vi "Estimate All Positions - Swarm Method (copy).vi"(0 "TagArray In":refnum<class "Tag.lvclass">[](array[class]), 1 "AllTagDistancesArray":T2(array[cluster]), 2 "AltTDA":T2(array[cluster]), 3 "Werkpunten":T5(array[cluster]), 5 "AnchorsArray":refnum<class "Anchor.lvclass">[](array[class]), 7 "error in (no error)":errorcluster) -> (13 "error out":errorcluster, 15 "Solution Vector":dbl[](array[numeric]) format="%.2f", 17 "SwarmOutputArray":T4(array[cluster]))   [LabVIEW 2014]
uses:
  Tag.lvclass
  Anchor/Anchor.lvclass
  <vilib>/Analysis/Matrix/Datatypes/RealMatrix.ctl
  <vilib>/Analysis/baseanly.llb/Matrix Type of Inverse Matrix.ctl
  <vilib>/Analysis/7linalg.llb/Solve Linear Equations (single right hand).vi
  <vilib>/Analysis/baseanly.llb/Solve Linear Equations By Cholesky.vi
  <vilib>/Analysis/baseanly.llb/Real Matrix to Compact Array.vi
  <vilib>/Analysis/baseanly.llb/Real Compact Tri-Matrix Linear Eqs.vi
  <vilib>/Analysis/Matrix/Numeric/Conversions/Array To Matrix - RA2.vi
  <vilib>/Analysis/7linalg.llb/Solve Linear Eqs (General).vi
  <vilib>/Analysis/7linalg.llb/Solve Linear Eqs (Gen, single right hand).vi
  <vilib>/Analysis/NI_AALPro.lvlib
  <vilib>/Analysis/NI_AALBase.lvlib
  <vilib>/Analysis/Matrix/NI_Matrix.lvlib
panel:
  out "fSwarmOutputArray":T1(array[cluster])
  out "RealSolutionVector":dbl[](array[numeric])
  out "Solution Vector AnchorToTag":dbl[](array[numeric]) format="%.2f"
  out "Solution Vector TagToTag":dbl[](array[numeric]) format="%.2f"
  out "Known Vector 3":T3
  out "Known Vector 2":T3
  out "Known Vector 1":T3
  out "Input Matrix 2":T3
  out "Input Matrix 1":T3
  out "Results Real":T3
  out "Input Matrix 3":T3
  out "# tags":i32=22
  out "Tag To":i32
  out "TagIDFrom":dbl format="%.2f"
  # "Output Indicators"
  # "Input Controls"
  # "Error Control"
  # "Error Indicator"
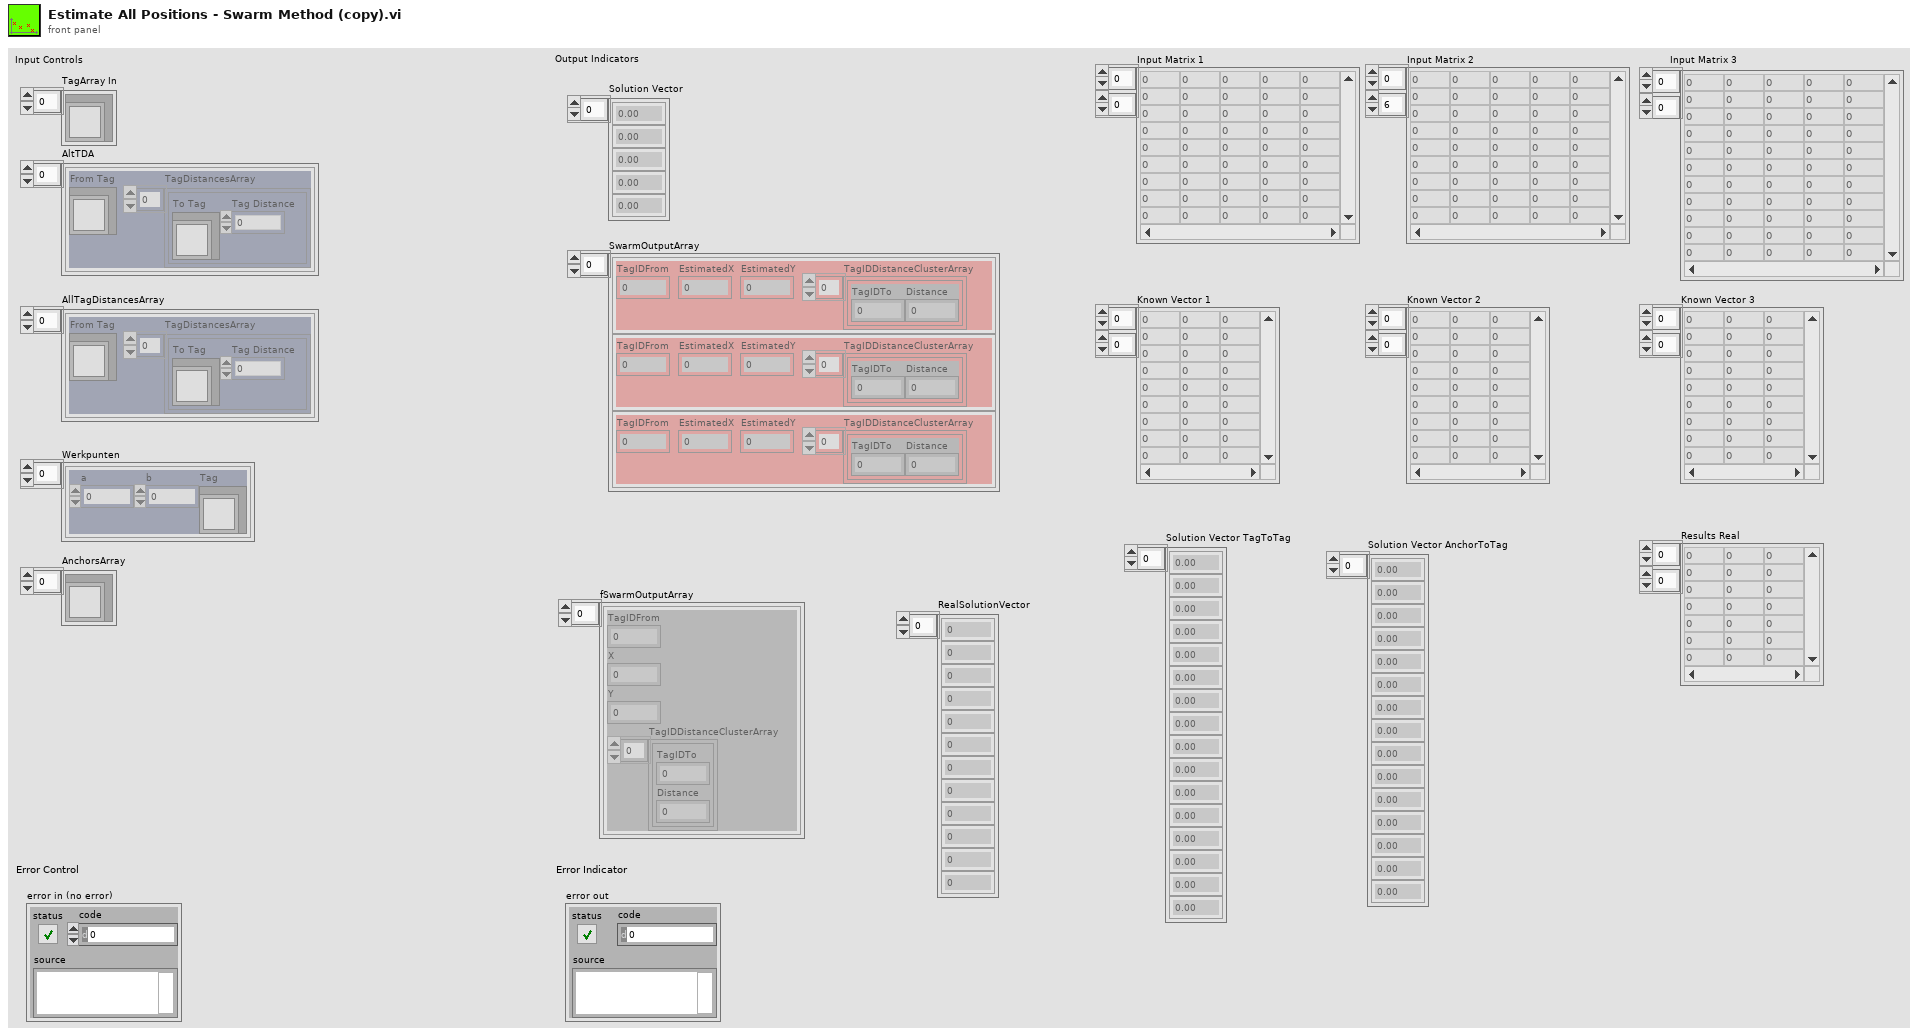
[diagram p1: front panel]
types:
  T1 = cluster{"TagIDFrom":dbl, "X":dbl, "Y":dbl, "TagIDDistanceClusterArray":cluster{"TagIDTo":dbl, "Distance":dbl}[]}[]
  T2 = cluster{"From Tag":refnum<class "Tag.lvclass">, "TagDistancesArray":cluster{"To Tag":refnum<class "Tag.lvclass">, "Tag Distance":dbl}[]}[]
  T3 = typedef "NI_Matrix.lvlib/RealMatrix.ctl" = dbl[][]
  T4 = cluster{"TagIDFrom":dbl, "EstimatedX":dbl, "EstimatedY":dbl, "TagIDDistanceClusterArray":cluster{"TagIDTo":dbl, "Distance":dbl}[]}[]
  T5 = cluster{"a":dbl, "b":dbl, "Tag":refnum<class "Tag.lvclass">}[]
  T6 = typedef "NI_AALBase.lvlib/Matrix Type of Inverse Matrix.ctl" = enum32{"General", "Positive Definite", "Lower Triangular", "Upper Triangular"}
  T7 = cluster{"From Tag":refnum<class "Tag.lvclass">, "TagDistancesArray":cluster{"To Tag":refnum<class "Tag.lvclass">, "Tag Distance":dbl}[]}
  T8 = cluster{"To Tag":refnum<class "Tag.lvclass">, "Tag Distance":dbl}[]
  T9 = cluster{"To Tag":refnum<class "Tag.lvclass">, "Tag Distance":dbl}
  T10 = cluster{"a":dbl, "b":dbl, "Tag":refnum<class "Tag.lvclass">}
  T11 = cluster{"TagID":dbl, dbl, dbl, "TagIDDistanceClusterArray":cluster{"TagIDTo":dbl, "Distance":dbl}[]}
  T12 = cluster{"TagID":dbl, "X":dbl, "Y":dbl, "TagIDDistanceClusterArray":cluster{"TagIDTo":dbl, "Distance":dbl}[]}[]
  T13 = cluster{"Tag.lvclass":refnum<class "Tag.lvclass">, "Distance":dbl}[]
  T14 = cluster{"TagIDFrom":dbl, "X":dbl, "Y":dbl, "TagIDDistanceClusterArray":cluster{"TagIDTo":dbl, "Distance":dbl}[]}
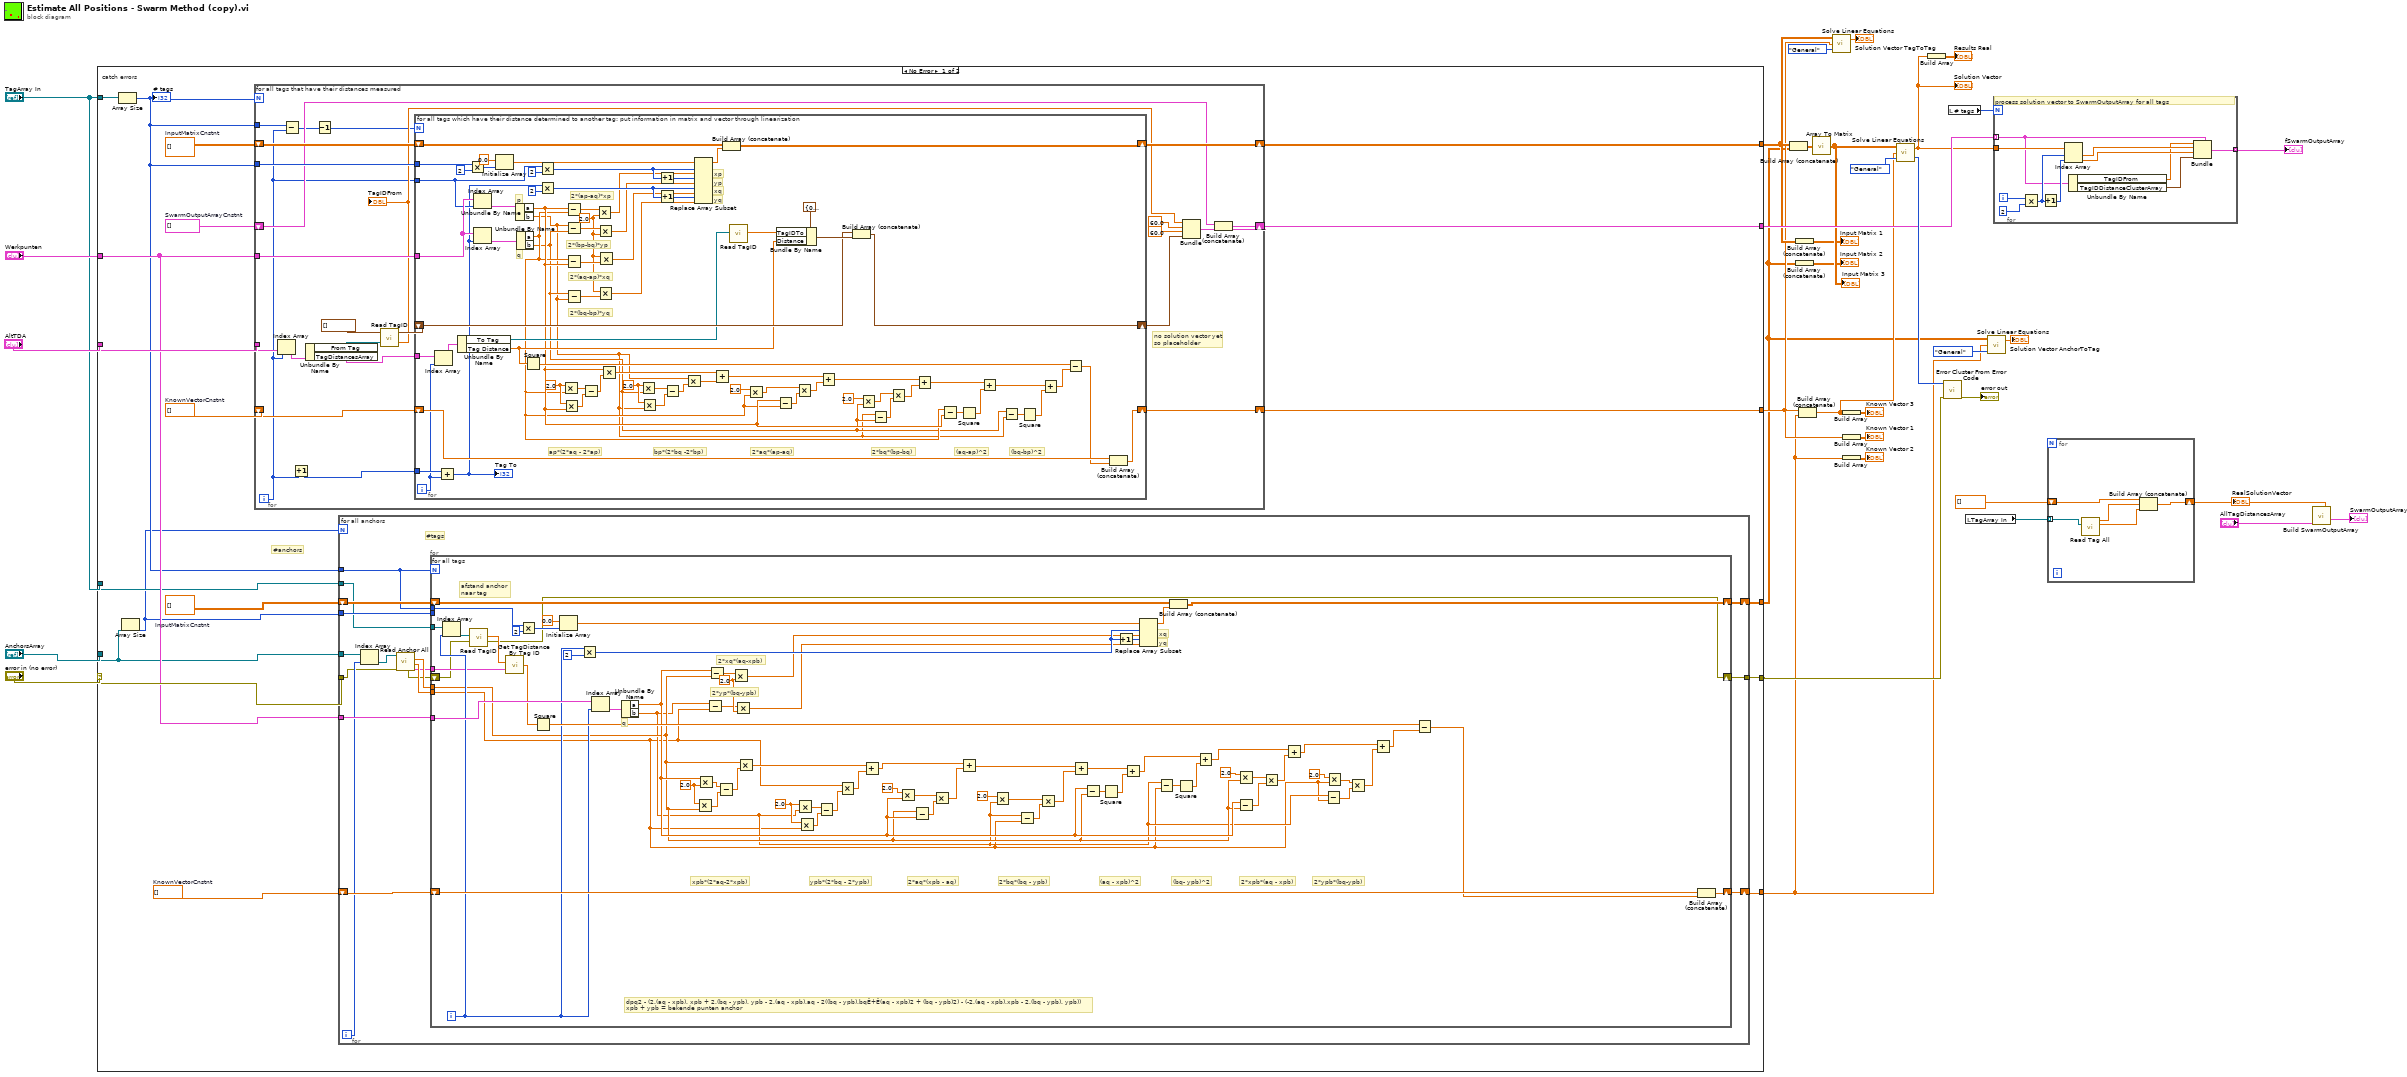
[diagram p0: block diagram]
diagram:
  n1 = case shown="No Error" "error in (no error)" {
    selector: "error in (no error)" -> [w48 w240]
    tunnel: [w53 _] -> w13
    tunnel: "Werkpunten" -> [w40 _]
    tunnel: "AnchorsArray" -> [w38 _]
    tunnel: [w51 _] -> w14
    tunnel: [w50 _] -> w9
    tunnel: [w49 _] -> w8
    tunnel: "TagArray In" -> [w43 _]
    tunnel: [w47 w240] -> w30
    tunnel: [w45 _] -> w28
    tunnel: "AltTDA" -> [w44 _]
    tunnel: "TagArray In" -> [w37 _]
    frame No Error {
      w41 = dbl[] []  # KnownVectorCnstnt
      w42 = dbl[][] []  # InputMatrixCnstnt
      w46 = T1 []  # SwarmOutputArrayCnstnt
      w52 = dbl[] []  # KnownVectorCnstnt
      w54 = dbl[][] []  # InputMatrixCnstnt
      # "#anchors"
      # "catch errors"
      n2 = Array Size(array=w43) -> (size(s)=w39:i32)
      "# tags" <- w39
      n3 = Array Size(array=w38) -> (size(s)=w36:i32)
      n4 = for {
        N: w39 -> [_]
        tunnel: w39 -> [w165]
        shift-right: [w162] -> w51
        shift-left: w54 -> [w163]
        tunnel: w39 -> [w161]
        tunnel: w40 -> [w160]
        shift-right: [w159] -> w53
        shift-left: w52 -> [w158]
        shift-right: [w153] -> w45
        shift-left: w46 -> [w154]
        tunnel: w44 -> [w147]
        i -> [w145]
        # "no solution vector yet\nso placeholder"
        # "for all tags that have their distances measured"
        n5 = Index Array "Index Array"(array=w147, index=w145) -> (element=w146:T7)
        n6 = Subtract(x=w165, y=w145) -> (x-y=w148:i32)
        n7 = Increment(x=w145) -> (x+1=w164:i32)
        n8 = Unbundle By Name(w146) -> ("From Tag"=w144:refnum<class "Tag.lvclass">, "TagDistancesArray"=w150:T8)
        n9 = Decrement(x=w148) -> (x-1=w143:i32)
        n10 = call "Read TagID.vi"("Tag in"=w144) -> ("TagID"=w149:dbl)  [unwired: 16 in, 2 out]
        "TagIDFrom" <- w149
        n11 = for {
          N: w143 -> [_]
          tunnel: w164 -> [w239]
          shift-right: [w238] -> w162
          shift-left: w163 -> [w232]
          tunnel: w161 -> [w234]
          tunnel: w160 -> [w216]
          tunnel: w145 -> [w215]
          shift-right: [w221] -> w159
          shift-left: w158 -> [w222]
          shift-right: [w217] -> w155
          shift-left: cluster{"TagIDTo":dbl, "Distance":dbl}[] [] ("TagIDDistanceClusterArray") -> [w218]
          tunnel: w150 -> [w211]
          i -> [w210]
          w192 = 2.0 ("x")
          w196 = 2.0 ("x")
          w199 = 2.0 ("y")
          # "(bq-bp)^2"
          # "(aq-ap)^2"
          # "2*bq*(bp-bq)"
          # "2*aq*(ap-aq)"
          # "bp*(2*bq -2*bp)"
          # "ap*(2*aq - 2*ap)"
          # "2*(bq-bp)*yq"
          # "2*(aq-ap)*xq"
          # "2*(bp-bq)*yp"
          # "2*(ap-aq)*xp"
          # "yq"
          # "xq"
          # "yp"
          # "xp"
          # "p"
          # "q"
          # "for all tags which have their distance determined to another tag: put information in matrix and vector through linearization"
          n12 = Index Array(array=w211, index=w210) -> (element=w209:T9)
          n13 = Add(x=w239, y=w210) -> (x+y=w212:i32)
          "Tag To" <- w212
          n14 = Unbundle By Name(w209) -> ("To Tag"=w213:refnum<class "Tag.lvclass">, "Tag Distance"=w208:dbl)
          n15 = Multiply(x=w234, y=2) -> (x*y=w237:i32)
          n16 = Index Array "Index Array"(array=w216, index=w215) -> (element=w230:T10)
          n17 = Index Array "Index Array"(array=w216, index=w212) -> (element=w229:T10)
          n18 = Initialize Array "Initialize Array"(0.0 ("element"), w237) -> (w231:dbl[])
          n19 = Unbundle By Name(w230) -> ("a"=w177:dbl, "b"=w169:dbl)
          n20 = Unbundle By Name(w229) -> ("a"=w176:dbl, "b"=w170:dbl)
          n21 = Square(x=w208) -> (x^2=w207:dbl)
          n22 = Multiply(x=w215, y=2) -> (x*y=w227:i32)
          n23 = Multiply(x=w212, y=2) -> (x*y=w224:i32)
          n24 = Multiply(x=w196, y=w176) -> (x*y=w197:dbl)
          n25 = Multiply(x=w196, y=w177) -> (x*y=w195:dbl)
          n26 = Subtract(x=w177, y=w176) -> (x-y=w206:dbl)
          n27 = Subtract(x=w169, y=w170) -> (x-y=w204:dbl)
          n28 = Subtract(x=w176, y=w177) -> (x-y=w202:dbl)
          n29 = Subtract(x=w170, y=w169) -> (x-y=w200:dbl)
          n30 = Subtract(x=w197, y=w195) -> (x-y=w194:dbl)
          n31 = Multiply(x=w206, y=w199) -> (x*y=w205:dbl)
          n32 = Multiply(x=w204, y=w199) -> (x*y=w203:dbl)
          n33 = Multiply(x=w199, y=w200) -> (x*y=w198:dbl)
          n34 = Multiply(x=w199, y=w202) -> (x*y=w201:dbl)
          n35 = Multiply(x=w177, y=w194) -> (x*y=w189:dbl)
          n36 = Multiply(x=w192, y=w170) -> (x*y=w193:dbl)
          n37 = Multiply(x=w192, y=w169) -> (x*y=w191:dbl)
          n38 = Increment(x=w227) -> (x+1=w226:i32)
          n39 = Increment(x=w224) -> (x+1=w223:i32)
          n40 = Subtract(x=w193, y=w191) -> (x-y=w190:dbl)
          n41 = Multiply(x=w169, y=w190) -> (x*y=w188:dbl)
          n42 = Replace Array Subset(array=w231, new element #1=w205, index #1=w227, new element #2=w203, index #2=w226, new element #3=w201, index #3=w224, new element #4=w198, index #4=w223) -> (w233:dbl[])
          n43 = Add(x=w189, y=w188) -> (x+y=w187:dbl)
          n44 = Build Array (concatenate)(w232, w233) -> (w238:dbl[][])
          n45 = call "Read TagID.vi"("Tag in"=w213) -> ("TagID"=w214:dbl)  [unwired: 16 in, 2 out]
          n46 = Multiply(x=2.0, y=w176) -> (x*y=w185:dbl)
          n47 = Bundle By Name(cluster=cluster{"TagIDTo":dbl, "Distance":dbl} {"TagIDTo"=0.0, "Distance"=0.0} ("TagIDDistanceCluster"), "TagIDTo"=w214, "Distance"=w208) -> (w219:cluster{"TagIDTo":dbl, "Distance":dbl})
          n48 = Subtract(x=w177, y=w176) -> (x-y=w183:dbl)
          n49 = Multiply(x=w185, y=w183) -> (x*y=w184:dbl)
          n50 = Add(x=w187, y=w184) -> (x+y=w179:dbl)
          n51 = Build Array (concatenate)(w218, w219) -> (w217:cluster{"TagIDTo":dbl, "Distance":dbl}[])
          n52 = Multiply(x=2.0, y=w170) -> (x*y=w181:dbl)
          n53 = Subtract(x=w169, y=w170) -> (x-y=w180:dbl)
          n54 = Multiply(x=w181, y=w180) -> (x*y=w178:dbl)
          n55 = Add(x=w179, y=w178) -> (x+y=w172:dbl)
          n56 = Subtract(x=w176, y=w177) -> (x-y=w175:dbl)
          n57 = Square(x=w175) -> (x^2=w173:dbl)
          n58 = Add(x=w172, y=w173) -> (x+y=w168:dbl)
          n59 = Subtract(x=w170, y=w169) -> (x-y=w174:dbl)
          n60 = Square(x=w174) -> (x^2=w171:dbl)
          n61 = Add(x=w168, y=w171) -> (x+y=w167:dbl)
          n62 = Subtract(x=w207, y=w167) -> (x-y=w166:dbl)
          n63 = Build Array (concatenate)(w222, w166) -> (w221:dbl[])
        }
        n64 = Bundle("TagID"=w149, 60.0, 60.0, "TagIDDistanceClusterArray"=w155) -> (w152:T11)  [unwired: 1 in]
        n65 = Build Array (concatenate)(w154, w152) -> (w153:T12)
      }
      n66 = for {
        N: w36 -> [_]
        tunnel: w39 -> [w55]
        tunnel: w40 -> [w71]
        tunnel: w36 -> [w70]
        tunnel: w38 -> [w62]
        shift-right: [w69] -> w50
        shift-left: w42 -> [w68]
        shift-right: [w66] -> w49
        shift-left: w41 -> [w67]
        tunnel: w48 -> [w59]
        tunnel: [w65] -> w47
        tunnel: w37 -> [w57]
        i -> [w63]
        # "#tags"
        # "for all anchors"
        n67 = Index Array(array=w62, index=w63) -> (element=w64:refnum<class "Anchor.lvclass">)
        n68 = call "Read Anchor All.vi"("error in (no error)"=w59, "Anchor in"=w64) -> ("TagDistanceArray"=w56:T13, "AnchorY"=w61:dbl, "AnchorX"=w60:dbl, "error out"=w58:errorcluster)  [unwired: 4 in, 2 out]
        n69 = for {
          N: w55 -> [_]
          tunnel: w71 -> [w142]
          tunnel: w70 -> [_]
          tunnel: w55 -> [w137]
          shift-right: [w141] -> w69
          shift-left: w68 -> [w140]
          shift-right: [w139] -> w66
          shift-left: w67 -> [w138]
          shift-right: [w118] -> w65
          shift-left: w58 -> [w119]
          tunnel: w61 -> [w74]
          tunnel: w60 -> [w80]
          tunnel: w57 -> [w123]
          tunnel: w56 -> [w120]
          i -> [w121]
          w106 = 2.0 ("x")
          w111 = 2.0 ("y")
          w115 = 2.0 ("y")
          # "2*ypb*(bq-ypb)"
          # "2*xpb*(aq - xpb)"
          # "(bq- ypb)^2"
          # "(aq - xpb)^2"
          # "2*bq*(bq - ypb)"
          # "2*aq*(xpb - aq)"
          # "ypb*(2*bq - 2*ypb)"
          # "xpb*(2*aq-2*xpb)"
          # "2*yp*(bq-ypb)"
          # "2*xq*(aq-xpb)"
          # "afstand anchor \nnaar tag"
          # "dpq2 - (2.(aq - xpb). xpb + 2.(bq - ypb). ypb - 2.(aq - xpb).aq - 2((bq - ypb).bqÊ+Ê(aq - xpb)2 + (bq - ypb)2) - (-2.(aq - xpb).xpb - 2.(bq - ypb). ypb))\nxpb + ypb = bekende punten anchor"
          # "yq"
          # "xq"
          # "q"
          # "for all tags"
          n70 = Index Array(array=w123, index=w121) -> (element=w122:refnum<class "Tag.lvclass">)
          n71 = call "Read TagID.vi"("Tag in"=w122, "error in (no error)"=w119) -> ("TagID"=w125:dbl, "error out"=w118:errorcluster)  [unwired: 15 in, 1 out]
          n72 = call "Get TagDistance By Tag ID.vi"("TagID"=w125, "TagDistanceArray"=w120) -> ("Distance"=w124:dbl)  [unwired: 13 in]
          n73 = Multiply(x=w137, y=2) -> (x*y=w129:i32)
          n74 = Square(x=w124) -> (x^2=w127:dbl)
          n75 = Initialize Array(0.0 ("element"), w129) -> (w133:dbl[])
          n76 = Multiply(x=w121, y=2) -> (x*y=w128:i32)
          n77 = Index Array(array=w142, index=w121) -> (element=w132:T10)
          n78 = Unbundle By Name(w132) -> ("a"=w81:dbl, "b"=w75:dbl)
          n79 = Multiply(x=w111, y=w80) -> (x*y=w109:dbl)
          n80 = Multiply(x=w81, y=w111) -> (x*y=w110:dbl)
          n81 = Subtract(x=w75, y=w74) -> (x-y=w114:dbl)
          n82 = Subtract(x=w81, y=w80) -> (x-y=w117:dbl)
          n83 = Subtract(x=w110, y=w109) -> (x-y=w112:dbl)
          n84 = Multiply(x=w117, y=w115) -> (x*y=w116:dbl)
          n85 = Multiply(x=w114, y=w115) -> (x*y=w113:dbl)
          n86 = Multiply(x=w80, y=w112) -> (x*y=w108:dbl)
          n87 = Multiply(x=w106, y=w75) -> (x*y=w107:dbl)
          n88 = Multiply(x=w106, y=w74) -> (x*y=w105:dbl)
          n89 = Subtract(x=w107, y=w105) -> (x-y=w104:dbl)
          n90 = Multiply(x=w74, y=w104) -> (x*y=w103:dbl)
          n91 = Add(x=w108, y=w103) -> (x+y=w102:dbl)
          n92 = Multiply(x=2.0, y=w81) -> (x*y=w100:dbl)
          n93 = Subtract(x=w80, y=w81) -> (x-y=w98:dbl)
          n94 = Multiply(x=w100, y=w98) -> (x*y=w99:dbl)
          n95 = Add(x=w102, y=w99) -> (x+y=w93:dbl)
          n96 = Multiply(x=2.0, y=w75) -> (x*y=w96:dbl)
          n97 = Subtract(x=w75, y=w74) -> (x-y=w95:dbl)
          n98 = Multiply(x=w96, y=w95) -> (x*y=w94:dbl)
          n99 = Add(x=w93, y=w94) -> (x+y=w91:dbl)
          n100 = Subtract(x=w81, y=w80) -> (x-y=w92:dbl)
          n101 = Square(x=w92) -> (x^2=w90:dbl)
          n102 = Increment(x=w128) -> (x+1=w130:i32)
          n103 = Add(x=w91, y=w90) -> (x+y=w89:dbl)
          n104 = Replace Array Subset(array=w133, new element #1=w116, index #1=w128, new element #2=w113, index #2=w130) -> (w134:dbl[])
          n105 = Subtract(x=w75, y=w74) -> (x-y=w88:dbl)
          n106 = Build Array (concatenate)(w140, w134) -> (w141:dbl[][])
          n107 = Square(x=w88) -> (x^2=w87:dbl)
          n108 = Add(x=w89, y=w87) -> (x+y=w86:dbl)
          n109 = Multiply(x=2.0, y=w80) -> (x*y=w84:dbl)
          n110 = Subtract(x=w81, y=w80) -> (x-y=w83:dbl)
          n111 = Multiply(x=w84, y=w83) -> (x*y=w82:dbl)
          n112 = Add(x=w86, y=w82) -> (x+y=w79:dbl)
          n113 = Subtract(x=w75, y=w74) -> (x-y=w73:dbl)
          n114 = Multiply(x=2.0, y=w74) -> (x*y=w76:dbl)
          n115 = Multiply(x=w76, y=w73) -> (x*y=w72:dbl)
          n116 = Add(x=w79, y=w72) -> (x+y=w78:dbl)
          n117 = Subtract(x=w127, y=w78) -> (x-y=w126:dbl)
          n118 = Build Array (concatenate)(w138, w126) -> (w139:dbl[])
        }
      }
    }
    frame Error {
    }
  }
  n119 = Build Array (concatenate)(w14, w9) -> (w24:dbl[][])
  n120 = Build Array (concatenate)(w14) -> (→"Input Matrix 1":T3)
  n121 = Build Array (concatenate)(w9) -> (→"Input Matrix 2":T3)
  n122 = Build Array (concatenate)(w13, w8) -> (w16:dbl[])
  n123 = call-poly <vilib>:"Array To Matrix.vi"("Real 2D Array"=w24) -> ("Real Matrix"=w23:T3)
  "Input Matrix 3" <- w23
  n124 = call-poly <vilib>:"Solve Linear Equations.vi"("matrix type"=Matrix_Type_of_Inverse_Matrix."General", "Known Vector"=w13, "Input Matrix"=w14) -> ("Solution Vector"=→"Solution Vector TagToTag":dbl[])  [unwired: 1 out]
  n125 = Build Array(w16) -> (→"Known Vector 3":T3)
  n126 = Build Array(w13) -> (→"Known Vector 1":T3)
  n127 = Build Array(w8) -> (→"Known Vector 2":T3)
  n128 = call-poly <vilib>:"Solve Linear Equations.vi"("matrix type"=Matrix_Type_of_Inverse_Matrix."General", "Known Vector"=w16, "Input Matrix"=w23) -> ("error"=w31:i32, "Solution Vector"=w22:dbl[])
  "Solution Vector" <- w22
  n129 = Build Array(w22) -> (→"Results Real":T3)
  n130 = call <vilib>:"Error Cluster From Error Code.vi"("error in (no error)"=w30, "error code (0)"=w31) -> ("error out"=→"error out":errorcluster)  [unwired: 7 in]
  n131 = local read "# tags"() -> (w27:i32)
  n132 = local read "TagArray In"() -> (w5:refnum<class "Tag.lvclass">[])
  n133 = call-poly <vilib>:"Solve Linear Equations.vi"("matrix type"=Matrix_Type_of_Inverse_Matrix."General", "Known Vector"=w8, "Input Matrix"=w9) -> ("Solution Vector"=→"Solution Vector AnchorToTag":dbl[])  [unwired: 1 out]
  n134 = for {
    N: w27 -> [_]
    tunnel: w28 -> [w243] mode=indexing
    tunnel: [w244] -> w1 mode=indexing
    tunnel: w22 -> [w251]
    i -> [w250]
    # "process solution vector to SwarmOutputArray for all tags"
    n135 = Multiply(x=w250, y=2) -> (x*y=w248:i32)
    n136 = Increment(x=w248) -> (x+1=w247:i32)
    n137 = Index Array(array=w251, index #1=w248, index #2=w247) -> (element #1=w246:dbl, element #2=w245:dbl)
    n138 = Unbundle By Name(w243) -> ("TagIDFrom"=w242:dbl, "TagIDDistanceClusterArray"=w241:cluster{"TagIDTo":dbl, "Distance":dbl}[])
    n139 = Bundle(cluster=w243, "TagIDFrom"=w242, "X"=w246, "Y"=w245, "TagIDDistanceClusterArray"=w241) -> (w244:T14)
  }
  "fSwarmOutputArray" <- w1
  n140 = for {
    shift-right: [w255] -> w4
    shift-left: dbl[] [] ("RealSolutionVector") -> [w256]
    tunnel: w5 -> [w254] mode=indexing
    n141 = call "Read Tag All.vi"("Tag.lvclass"=w254) -> ("TagY"=w252:dbl, "TagX"=w253:dbl)  [unwired: 5 in, 4 out]
    n142 = Build Array (concatenate)(w256, w253, w252) -> (w255:dbl[])
  }
  "RealSolutionVector" <- w4
  n143 = call "Build SwarmOutputArray.vi"("AllTagDistancesArray"="AllTagDistancesArray", "Solution Vector"=w4) -> ("SwarmOutputArray"=→"SwarmOutputArray":T4)  [unwired: 9 in]
